vi "Victory Message.vi"(11 "MyTeam in":refnum<class "MyTeam.lvclass">) -> (2 "Victory Message":string)   [LabVIEW 2020, in "Galaxy.lvlib" / "MyTeam.lvclass"]
uses:
  MyTeam.lvclass
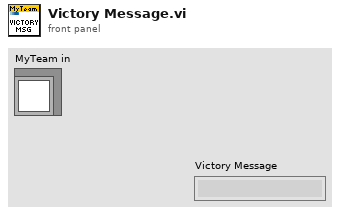
[diagram p1: front panel]
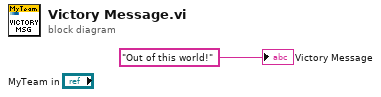
[diagram p0: block diagram]
diagram:
  "Victory Message" <- "Out of this world!" ("Victory Message")
